vi "SyncTest.vi"() -> ()   [LabVIEW 2014]
uses:
  dll/LabviewDllTest2_ParallelRunning.dll
panel:
  out "x+1":i32
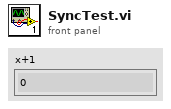
[diagram p1: front panel]
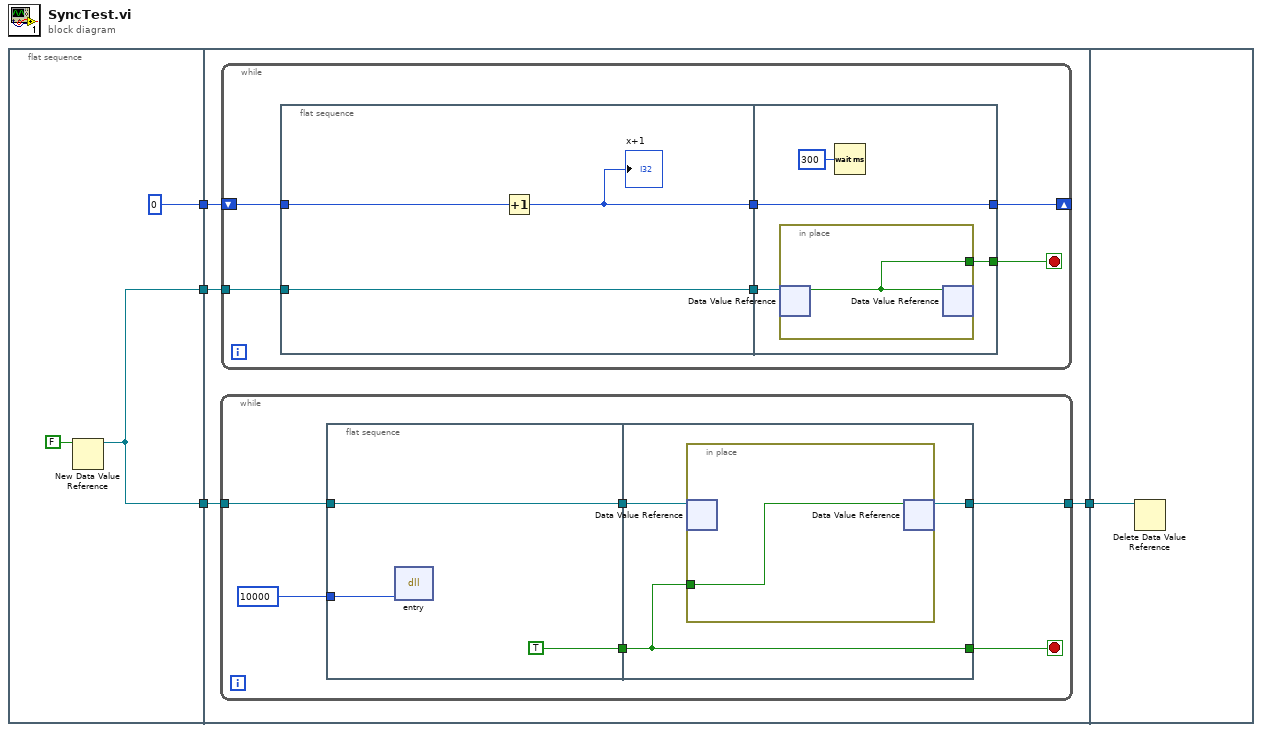
[diagram p0: block diagram]
diagram:
  n1 = flat-sequence {
    tunnel: [0] -> w4
    tunnel: [w5] -> w3
    tunnel: [w5] -> w2
    tunnel: w4 -> [w11]
    tunnel: w3 -> [w9]
    tunnel: w2 -> [w10]
    tunnel: [w8] -> w1
    tunnel: w1 -> [w39]
    frame #0 {
      n2 = New Data Value Reference(data value=FALSE) -> (data value reference=w5:refnum<data-value>)  [unwired: 1 in, 1 out]
    }
    frame #1 {
      n3 = while {
        tunnel: w10 -> [w13]
        tunnel: [w12] -> w8
        stop <- w16 stop-if-true
        n4 = flat-sequence {
          tunnel: 10000 -> [w20]
          tunnel: [TRUE] -> w15
          tunnel: [w18] -> w14
          tunnel: w13 -> [w18]
          tunnel: [w22] -> w16
          tunnel: w15 -> [w22]
          tunnel: w14 -> [w23]
          tunnel: [w21] -> w12
          frame #0 {
            n5 = dll-call lib="C:/Users/DrippySummer/Documents/LabVIEW Data/SavaData/MultiChannelKeithley/dll/LabviewDllTest2_ParallelRunning.dll" fn="entry"("pInput"=w20) -> ()  [unwired: 5 in, 2 out]
          }
          frame #1 {
            n6 = in-place {
              in-place-border: w22 -> [w24]
              n7 = in-place-dvr #1(w23) -> ()  [unwired: 2 out]
              n8 = in-place-dvr #1(w24) -> (w21:refnum<data-value>)  [unwired: 1 out]
            }
          }
        }
      }
      n9 = while {
        shift-right: [w28] -> _
        shift-left: w11 -> [w30]
        tunnel: w9 -> [w27]
        stop <- w25 stop-if-true
        n10 = flat-sequence {
          tunnel: w30 -> [w33]
          tunnel: [w32] -> w29
          tunnel: w27 -> [w31]
          tunnel: [w31] -> w26
          tunnel: w29 -> [w37]
          tunnel: [w37] -> w28
          tunnel: w26 -> [w35]
          tunnel: [w34] -> w25
          frame #0 {
            n11 = Increment(x=w33) -> (x+1=w32:i32)
            "x+1" <- w32
          }
          frame #1 {
            n12 = in-place {
              in-place-border: [w38] -> w34
              n13 = in-place-dvr #2(w35) -> (w38:bool)  [unwired: 1 out]
              n14 = in-place-dvr #2(w38) -> ()  [unwired: 2 out]
            }
            n15 = Wait (ms)(milliseconds to wait=u32 300) -> ()  [unwired: 1 out]
          }
        }
      }
    }
    frame #2 {
      n16 = Delete Data Value Reference(data value reference=w39) -> ()  [unwired: 1 in, 2 out]
    }
  }
